vi "InsertData.vi"() -> ()   [LabVIEW 2020]
uses:
  <vilib>/addons/database/NI_Database_API.lvlib
panel:
  in  "error in (no error)":errorcluster
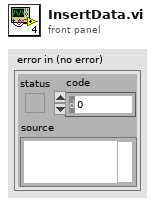
[diagram p1: front panel]
types:
  T1 = typedef "NI_Database_API.lvlib/Conn ObjectReference.ctl" = refnum<k1>
  T2 = cluster{"Name":string, "Password":string, "GroupID":i32, "Date/time":timestamp, "RawData":cluster{"Element1":i32, "String":string}}
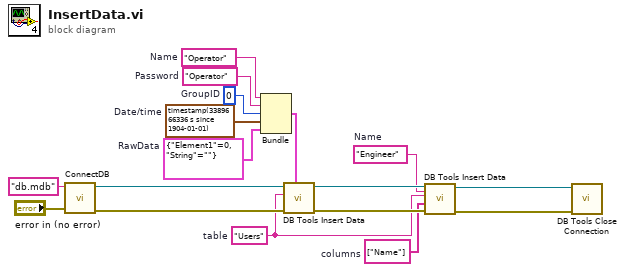
[diagram p0: block diagram]
diagram:
  w10 = timestamp(3389666336.917968 s since 1904-01-01)  # Date/time
  w1 = "Engineer"  # Name
  w4 = string[] ["Name"]  # columns
  w9 = cluster{"Element1":i32, "String":string} {"Element1"=0, "String"=""}  # RawData
  w11 = 0  # GroupID
  w12 = "Operator"  # Password
  w13 = "Operator"  # Name
  w5 = "Users"  # table
  n1 = call "ConnectDB.vi"("error in (no error)"="error in (no error)", "Filename"="db.mdb") -> ("error out"=w14:errorcluster, "DB Conn"=w15:T1)  [unwired: 8 in]
  n2 = Bundle("Name"=w13, "Password"=w12, "GroupID"=w11, "Date/time"=w10, "RawData"=w9) -> (w8:T2)  [unwired: 1 in]
  n3 = call <vilib>:"DB Tools Insert Data.vi"("data"=w8, "error in (no error)"=w14, "table"=w5, "connection reference"=w15) -> ("error out"=w7:errorcluster, "connection reference out"=w6:T1)  [unwired: 6 in]
  n4 = call <vilib>:"DB Tools Insert Data.vi"("data"=w1, "error in (no error)"=w7, "columns"=w4, "table"=w5, "connection reference"=w6) -> ("error out"=w3:errorcluster, "connection reference out"=w2:T1)  [unwired: 5 in]
  n5 = call <vilib>:"DB Tools Close Connection.vi"("error in (no error)"=w3, "connection reference"=w2) -> ()  [unwired: 5 in, 1 out]
